vi "Read Maximum Step Rate.vi"(11 "StepperMotor in":refnum<class "StepperMotor.lvclass">) -> (2 "Maximum Step Rate":dbl[unit]=5000000.0 min=10000.0 max=5000000.0, 3 "StepperMotor out":refnum<class "StepperMotor.lvclass">)   [LabVIEW 2013, in "StepperMotor.lvlib" / "StepperMotor.lvclass"]
uses:
  <userlib>/Common/Devices/StepperMotor/StepperMotor/StepperMotor.lvclass
  <userlib>/Common/Devices/StepperMotor/StepperMotor/StepperMotor.lvclass/StepperMotor.ctl
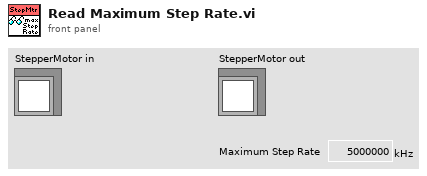
[diagram p1: front panel]
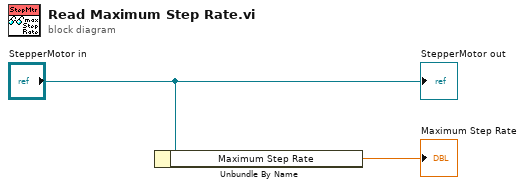
[diagram p0: block diagram]
diagram:
  n1 = Unbundle By Name("StepperMotor in") -> ("Maximum Step Rate"=→"Maximum Step Rate":dbl[unit])
  "StepperMotor out" <- "StepperMotor in"
